vi "PV Packet 2.vi"(11 "HEX Data (U8) in":u8[](array[numeric])) -> (3 "PV Data 2":string[](array[string]))   [LabVIEW 2023]
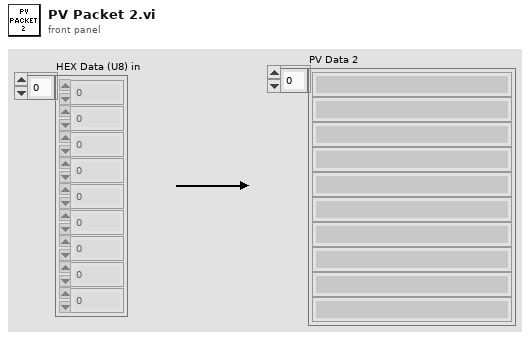
[diagram p1: front panel]
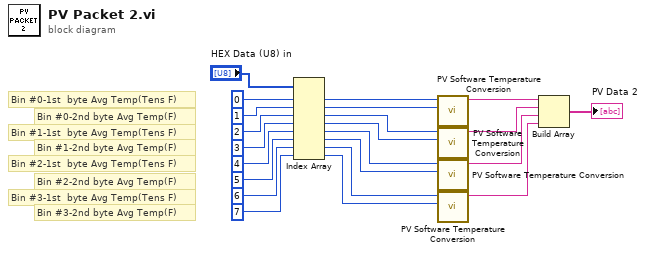
[diagram p0: block diagram]
diagram:
  # "Bin #3-2nd byte Avg Temp(F)"
  # "Bin #3-1st  byte Avg Temp(Tens F)"
  # "Bin #2-2nd byte Avg Temp(F)"
  # "Bin #2-1st  byte Avg Temp(Tens F)"
  # "Bin #1-2nd byte Avg Temp(F)"
  # "Bin #1-1st  byte Avg Temp(Tens F)"
  # "Bin #0-2nd byte Avg Temp(F)"
  # "Bin #0-1st  byte Avg Temp(Tens F)"
  n1 = Index Array(array="HEX Data (U8) in", index #1=0 ("disabled index (col)"), index #2=1 ("disabled index (col)"), index #3=2 ("disabled index (col)"), index #4=3 ("disabled index (col)"), index #5=4 ("disabled index (col)"), index #6=5 ("disabled index (col)"), index #7=6 ("disabled index (col)"), index #8=7 ("disabled index (col)")) -> (element #1=w17:u8, element #2=w16:u8, element #3=w15:u8, element #4=w14:u8, element #5=w13:u8, element #6=w12:u8, element #7=w11:u8, element #8=w10:u8)
  n2 = call "PV Software Temperature Conversion.vi"("HEX Data (Byte 2)"=w16, "HEX Data (Byte 1)"=w17) -> ("Temperature (F)"=w18:string)  [unwired: 9 in]
  n3 = call "PV Software Temperature Conversion.vi"("HEX Data (Byte 2)"=w14, "HEX Data (Byte 1)"=w15) -> ("Temperature (F)"=w19:string)  [unwired: 9 in]
  n4 = call "PV Software Temperature Conversion.vi"("HEX Data (Byte 2)"=w12, "HEX Data (Byte 1)"=w13) -> ("Temperature (F)"=w20:string)  [unwired: 9 in]
  n5 = call "PV Software Temperature Conversion.vi"("HEX Data (Byte 2)"=w10, "HEX Data (Byte 1)"=w11) -> ("Temperature (F)"=w21:string)  [unwired: 9 in]
  n6 = Build Array(w18, w19, w20, w21) -> (→"PV Data 2":string[])
